vi "Soft_Robot_Model_ffwd.vi"() -> ()   [LabVIEW 2015]
uses:
  <vilib>/addons/Control Design/_Stochastic Systems/Stochastic Systems.llb/Stochastic Systems SubVIs/cd_Stochastic State-Space Model.ctl
  <vilib>/addons/Control Design/_Model Construction/Model Typedefs.llb/CD State Space Model (MIMO).ctl
  <vilib>/addons/Control Design/_Model Construction/Model Typedefs.llb/CD General Elements.ctl
  <vilib>/addons/Control Design/_Stochastic Systems/Stochastic Systems.llb/Stochastic Systems SubVIs/cd_Second-Order Statistics Noise Model.ctl
  <vilib>/Analysis/Matrix/Datatypes/RealMatrix.ctl
  <vilib>/addons/Control Design/_Stochastic Systems/Stochastic Systems.llb/CD CtoD Stochastic Model.ctl
  <vilib>/Analysis/7linalg.llb/Eigenvalue and Vectors Output Option.ctl
  <vilib>/Platform/TimedLoop/XDataNode/timing_clust.ctl
  <vilib>/Platform/TimedLoop/XDataNode/nitl_modes.ctl
  <vilib>/Platform/TimedLoop/XDataNode/wakeup.ctl
  <vilib>/Simulation/Scripting/Companion Diagram/SimConfigNode/SimParams.ctl
  <vilib>/Simulation/Scripting/Companion Diagram/SimConfigNode/_simSolvers.ctl
  <vilib>/Simulation/Implementation/Shared/SIMSCR Execution Mode.ctl
  <vilib>/Simulation/Param Hierarchy/Typedefs/SIMPH Param Control Actions.ctl
  <vilib>/Simulation/Implementation/Shared/NILVSim_ParamChanged.vi
  <vilib>/Simulation/Implementation/Shared/NILVSim_FinishedLate.vi
  <vilib>/Simulation/Implementation/Shared/NILVSIM_BeginStep.vi
  <vilib>/Simulation/SignalArithmetic/Implementation/NILVSim Gain.llb/SIM Gain (scalar).vi
  <vilib>/Simulation/Implementation/Shared/NILVSim_Manager.vi
  <vilib>/Utility/error.llb/Clear Errors.vi
  <vilib>/Simulation/Implementation/Shared/NILVSim_FinalizeModel.vi
  <vilib>/addons/Control Design/_Stochastic Systems/Stochastic Systems.llb/CD Construct Stochastic Model (Numeric).vi
  <vilib>/Analysis/7linalg.llb/Create Special Real Matrix.vi
  <vilib>/addons/Control Design/_Stochastic Systems/Stochastic Systems.llb/CD Construct Noise Model (Numeric).vi
  <vilib>/Analysis/7linalg.llb/Real Eigenvalues and Vectors.vi
  <vilib>/addons/Control Design/_State Feedback Control/State Feedback Control.llb/State Feedback Control SubVis/cd_Linear Quadratic Regulator.vi
  <vilib>/FPGAPlugInAG/myRIO-1900/niLvFpga_Open_myRIO-1900.vi
  <vilib>/rvi/interface/common/dynamic/niFpgaDynamicAddResources.vi
  <vilib>/Utility/error.llb/Error Cluster From Error Code.vi
  <vilib>/rvi/errors/niLvFpgaAdjustHostInterfaceError.vi
  <vilib>/FPGAPlugInAG/Dynamic/niLvFpga_Close_Dynamic.vi
  <vilib>/Simulation/Implementation/Shared/SIM Unbundle Sim Info.vi
  <vilib>/Simulation/Implementation/Shared/SIMSH Read Queue.vi
  <vilib>/Simulation/Implementation/Shared/NILVSim_Initialize.vi
  <vilib>/Utility/file.llb/Write Delimited Spreadsheet.vi
  <vilib>/Utility/file.llb/Write Delimited Spreadsheet (I64).vi
  <vilib>/Utility/file.llb/Write Delimited Spreadsheet (DBL).vi
  <vilib>/addons/Control Design/_Time Response Analysis/Time Response.llb/CD Impulse Response.vi
  <vilib>/addons/Control Design/_Time Response Analysis/Time Response.llb/Time Response subVI/cd_Impulse Response (State-Space).vi
  <vilib>/addons/Control Design/_Time Response Analysis/Time Response.llb/CD Step Response.vi
  <vilib>/addons/Control Design/_Time Response Analysis/Time Response.llb/Time Response subVI/cd_Step Response (State-Space).vi
  <vilib>/Simulation/Utility/Implementation/NILVSim Get Time and IsAcceptedStep.vi
  <vilib>/Simulation/Estimation/Implementation/NILVSim Discrete Kalman Filter.llb/SIM Disc KF Pred and Corr with Pred Gain with Checking Indirect Distributor Sim.vi
  <vilib>/addons/Control Design/_Implementation/CD State Feedback Controller.vi
  <vilib>/addons/Control Design/_Implementation/CD State Feedback Controller (Multiple Outputs).vi
  <vilib>/Simulation/Estimation/Implementation/NILVSim Discrete Kalman Filter.llb/SIM Disc KF Pred and Corr with Pred Gain with Checking Indirect Collector Sim.vi
  <vilib>/Simulation/Implementation/Shared/NILVSim_GetModelError.vi
  <vilib>/Simulation/Implementation/Shared/SIM Bundle Sim Info.vi
  <vilib>/Platform/TimedLoop/XDataNode/XDataNode.xnode
  <vilib>/rvi/interface/nirviOpenFPGA/nirviOpenFPGA.xnode
  FPGA Bitfiles/ACC20115_FPGATarget_CurrentControlle_W-6n2rsGK8k.lvbitx
  Misc/Current Controller.vi
  <vilib>/rvi/interface/nirviReadWriteControl/nirviReadWriteControl.xnode
  <vilib>/rvi/interface/nirviCloseFPGA/nirviCloseFPGA.xnode
  <vilib>/Simulation/Scripting/Companion Diagram/SimConfigNode/SimDog.xnode
  <vilib>/Simulation/Implementation/XNodeFramework/SimXNode/SimX.xnode
  <vilib>/addons/Control Design/_State Feedback Control/NI_CD_State Feedback Control.lvlib
  <vilib>/Analysis/NI_AALPro.lvlib
  <vilib>/Platform/TimedLoop/XDataNode/XDNodeRunTimeDep.lvlib
  <vilib>/rvi/interface/Simulation/niFpgaSimulationCallBeginRW.vi
  <vilib>/addons/Control Design/_Stochastic Systems/NI_CD_Stochastic Systems.lvlib
  <vilib>/addons/Control Design/_State-Space Analysis/NI_CD_State-Space Analysis.lvlib
  NiFpgaLv.dll
  <vilib>/addons/Control Design/_Implementation/NI_CD_Implementation.lvlib
  <vilib>/addons/Control Design/_Time Response Analysis/NI_CD_Time Response.lvlib
  <vilib>/Simulation/Estimation/Implementation/NILVSim Discrete Kalman Filter.llb/SIM Disc KF Pred and Corr with Pred Gain with Checking Indirect Sim.vi
  <vilib>/Simulation/Implementation/Shared/NI_SIM_Implementation.lvlib
  <vilib>/addons/Control Design/_Model Construction/NI_LinSys_Model Typedefs.lvlib
  <vilib>/Analysis/Matrix/NI_Matrix.lvlib
panel:
  out "Error":errorcluster
  in  "Tab Control":T1(tab)
  out "Valve Current (mA)":dbl(graph)
  out "Kinect Fusion":dbl(graph)
  in  "Current (mA)":i32
  out "Plant Output and KF estimation":dbl[][](graph)=[[694.135, 693.2125685090368]]
  out "KF Predictor Gain L(k)":dbl[][](array[numeric])=[[1.0]] format="%#.6g"
  out "KF Gain M(k)":dbl[][](array[numeric]) format="%#.6g"
  in  "Stop":bool
  out "LQR Eigenvalues":cdb[](array[numeric]) format="%.5f"
  out "P(k+1|k)":dbl[][](array[numeric])
  out "P(k|k)":dbl[][](array[numeric])
  out "LQR Q Eig Vals":cdb[](array[numeric])
  out "LQR R Eig Val":cdb[](array[numeric])
  out "Optimal LQR Gains":dbl[][](array[numeric])
  out "Control Action":dbl
  out "Controllable?":bool
  out "Stable?":bool
  out "Detectable?":bool
  out "Observable?":bool
  out "LQR Q Matrix":T2
  out "LQR R Matrix":T2
  out "FPGA Overflow?":bool
  in  "SP (mm)":dbl(knob)=641.7660208643815 scale=670.0..695.0
  out "Local Kalman Filters & Central Site Fusion":dbl[][](graph)
  out "Stochastic SS Model":T3={"Sampling Time (s)"=0.0, "G"=[], "B"=[[-1.71e-07], [6.47e-07]], "A"=[], "C"=[], "D"=[], "H"=[]} {"H" format="%#.2g"; "D" format="%#.2g"; "C" format="%#.2g"; "A" format="%#.2g"; "B" format="%#.2g"; "G" format="%#.2g"; "Sampling Time (s)" format="%.2f"}
  out "Deterministic SS Model":T4={"properties"={"Model name"="", "Input names"=[], "Output names"=[], "Input Delays"=[], "Output Delays"=[], "Sampling Time"=0.0, "Notes"=""}, "A"=[], "B"=[[-1.706e-07], [6.469e-07]], "C"=[], "D"=[], "StateNames"=[], "Transport Delay"=[]} {"Transport Delay" format="%.2f"; "D" format="%#.2g"; "C" format="%#.2g"; "B" format="%#.2g"; "A" format="%#.2g"; "properties"."Sampling Time" format="%#.6p"; "properties"."Output Delays" format="%.4f"; "properties"."Input Delays" format="%.4f"}
  out "DAC Loop Error":errorcluster
  out "LQR Error":errorcluster
  out "KF Noise Model":T6 {"N" format="%#.2g"; "R" format="%#.2g"; "E{v}" format="%#.2g"; "E{w}" format="%#.2g"; "Q" format="%#.2g"}
  out "FPGA Loop Error":errorcluster
  out "KF Model Error":errorcluster
  out "UDP Loop Error":errorcluster
  out "Step Response Graph":cluster{"time":dbl[], dbl[]}[](graph)=[{"time"=[0.0, 0.1, 0.2, 0.30000000000000004, 0.4, 0.5, 0.6000000000000001, 0.7000000000000001, 0.8, 0.9, 1.0, 1.1, 1.2000000000000002, 1.3, 1.4000000000000001, 1.5, 1.6, 1.7000000000000002, 1.8, 1.9000000000000001, 2.0, 2.1, 2.2, 2.3000000000000003, 2.4000000000000004, 2.5, 2.6, 2.7, 2.8000000000000003, 2.9000000000000004, 3.0, 3.1, 3.2, 3.3000000000000003, 3.4000000000000004, 3.5, 3.6, 3.7, 3.8000000000000003, 3.9000000000000004, 4.0, 4.1000000000000005, 4.2, 4.3, 4.4, 4.5, 4.6000000000000005, 4.7, 4.800000000000001, 4.9, 5.0, 5.1000000000000005, 5.2, 5.300000000000001, 5.4, 5.5, 5.6000000000000005, 5.7, 5.800000000000001, 5.9, 6.0, 6.1000000000000005, 6.2, 6.300000000000001, 6.4, 6.5, 6.6000000000000005, 6.7, 6.800000000000001, 6.9, 7.0, 7.1000000000000005, 7.2, 7.300000000000001, 7.4, 7.5, 7.6000000000000005, 7.7, 7.800000000000001, 7.9, 8.0], [0.0, 0.0004663473208612627, 0.0017296930483795164, 0.0035885524413313812, 0.00585108885158747, 0.008342022204108804, 0.010907538001557412, 0.013418337758795643, 0.01577103010603519, 0.017888100567384182, 0.019716719021094366, 0.02122664935211373, 0.022407518377011763, 0.02326568343598631, 0.02382091276348735, 0.024103062386256875, 0.024148900146291487, 0.023999193507947617, 0.02369614475738421, 0.023281226369499006, 0.02279344169187109, 0.022268012342287972, 0.021735474206151545, 0.021221148763839872, 0.020744945570676618, 0.020321444775591793, 0.01996020519209235, 0.019666243132932183, 0.01944062944497821, 0.019281156374667745, 0.019183031510994153, 0.01913956258079366, 0.019142803850451515, 0.019184141922185993, 0.01925480547445023, 0.01934628972900578, 0.019450691946355205, 0.019560958936806403, 0.019671051366119408, 0.01977603252338114, 0.019872091237783975, 0.01995650984687708, 0.020027588622327185, 0.02008453795668775, 0.020127349020610013, 0.02015665263024424, 0.020173574831124263, 0.02017959631108057, 0.02017642129264157, 0.02016586010332895, 0.020149728243942358, 0.02012976351919565, 0.020107561696361465, 0.0200845302370225, 0.0200618589138676, 0.02004050557782586, 0.020021194971562285, 0.020004428277976674, 0.01999050102686616, 0.019979527036564866, 0.0199714662161444, 0.019966154273690646, 0.019963332644441115, 0.019962677248304108, 0.019963824991160707, 0.019966397222957007, 0.019970019645588307, 0.019974338415697335, 0.019979032405429503, 0.019983821764274674, 0.01998847306610796, 0.01999280142814749, 0.019996670055101227, 0.019999987695808956, 0.020002704505559007, 0.020004806789810977, 0.02000631106930135, 0.020007257857379883, 0.020007705482562522, 0.0200077242268862, 0.02000739098734998]}]
  out "Impulse Response":cluster{"time":dbl[], dbl[]}[](graph)=[{"time"=[0.0, 0.1, 0.2, 0.30000000000000004, 0.4, 0.5, 0.6000000000000001, 0.7000000000000001, 0.8, 0.9, 1.0, 1.1, 1.2000000000000002, 1.3, 1.4000000000000001, 1.5, 1.6, 1.7000000000000002, 1.8, 1.9000000000000001, 2.0, 2.1, 2.2, 2.3000000000000003, 2.4000000000000004, 2.5, 2.6, 2.7, 2.8000000000000003, 2.9000000000000004, 3.0, 3.1, 3.2, 3.3000000000000003, 3.4000000000000004, 3.5, 3.6, 3.7, 3.8000000000000003, 3.9000000000000004, 4.0, 4.1000000000000005, 4.2, 4.3, 4.4, 4.5, 4.6000000000000005, 4.7, 4.800000000000001, 4.9, 5.0, 5.1000000000000005, 5.2, 5.300000000000001, 5.4, 5.5, 5.6000000000000005, 5.7, 5.800000000000001, 5.9, 6.0, 6.1000000000000005, 6.2, 6.300000000000001, 6.4, 6.5, 6.6000000000000005, 6.7, 6.800000000000001, 6.9, 7.0, 7.1000000000000005, 7.2, 7.300000000000001, 7.4, 7.5, 7.6000000000000005, 7.7, 7.800000000000001, 7.9, 8.0], [0.0, 0.008988172215977587, 0.015941438633037666, 0.02091487162309135, 0.024042908393783827, 0.02551889757722494, 0.02557569478365717, 0.024467992676866855, 0.022456868580669295, 0.019796844996257237, 0.016725591461953054, 0.013456253705261323, 0.010172280017081137, 0.007024525658691236, 0.004130353039235721, 0.0015744064999214857, -0.0005892768149515742, -0.002334157452931432, -0.0036574068645988137, -0.004575736995437892, -0.005121104002831364, -0.005336502802076594, -0.005272025764550862, -0.004981315552097141, -0.004518500722641401, -0.003935664888301879, -0.0032808669235171064, -0.0025967016806585676, -0.001919368189106927, -0.0012781953978247278, -0.0006955639255905182, -0.0001871555662120171, 0.0002375401230830873, 0.0005745316131444697, 0.0008245089129275849, 0.0009919638112413014, 0.0010842980213564997, 0.0011109616697939839, 0.0010826555079039139, 0.0010106212985917036, 0.0009060364188353945, 0.0007795211078167689, 0.000640760178844977, 0.0004982355180431294, 0.00035906135961267507, 0.00022891114129368586, 0.0001120226402826769, 1.1266967989904443e-05, -7.17332656671379e-05, -0.00013645086398689086, -0.0001832792705777772, -0.0002133479298936649, -0.00022833790229576505, -0.0002303060085980187, -0.00022152389413133484, -0.00020433657074322872, -0.00018104328983030286, -0.0001538020745465803, -0.00012455793086593947, -9.499368500849999e-05, -6.650156442132397e-05, -4.0173044664881016e-05, -1.6804109357439747e-05, 3.087108111676786e-06, 1.9233341685522883e-05, 3.158477953815003e-05, 4.027189426429472e-05, 4.556687476968165e-05, 4.7845653868121716e-05, 4.755213725597536e-05, 4.516584913005334e-05, 4.117383523520003e-05, 3.6047319585871326e-05, 3.0223306623967816e-05, 2.4091062632339335e-05, 1.7983202024296476e-05, 1.2170946052935176e-05, 6.863011578249593e-06, 2.207522022942255e-06, -1.7036935523276584e-06, -4.8290401595337954e-06]}]
  out "Step and Impulse Response Plots":cluster{"time":dbl[], dbl[]}[](graph)=[{"time"=[0.0, 0.1, 0.2, 0.30000000000000004, 0.4, 0.5, 0.6000000000000001, 0.7000000000000001, 0.8, 0.9, 1.0, 1.1, 1.2000000000000002, 1.3, 1.4000000000000001, 1.5, 1.6, 1.7000000000000002, 1.8, 1.9000000000000001, 2.0, 2.1, 2.2, 2.3000000000000003, 2.4000000000000004, 2.5, 2.6, 2.7, 2.8000000000000003, 2.9000000000000004, 3.0, 3.1, 3.2, 3.3000000000000003, 3.4000000000000004, 3.5, 3.6, 3.7, 3.8000000000000003, 3.9000000000000004, 4.0, 4.1000000000000005, 4.2, 4.3, 4.4, 4.5, 4.6000000000000005, 4.7, 4.800000000000001, 4.9, 5.0, 5.1000000000000005, 5.2, 5.300000000000001, 5.4, 5.5, 5.6000000000000005, 5.7, 5.800000000000001, 5.9, 6.0, 6.1000000000000005, 6.2, 6.300000000000001, 6.4, 6.5, 6.6000000000000005, 6.7, 6.800000000000001, 6.9, 7.0, 7.1000000000000005, 7.2, 7.300000000000001, 7.4, 7.5, 7.6000000000000005, 7.7, 7.800000000000001, 7.9, 8.0], [0.0, 0.0004663473208612627, 0.0017296930483795164, 0.0035885524413313812, 0.00585108885158747, 0.008342022204108804, 0.010907538001557412, 0.013418337758795643, 0.01577103010603519, 0.017888100567384182, 0.019716719021094366, 0.02122664935211373, 0.022407518377011763, 0.02326568343598631, 0.02382091276348735, 0.024103062386256875, 0.024148900146291487, 0.023999193507947617, 0.02369614475738421, 0.023281226369499006, 0.02279344169187109, 0.022268012342287972, 0.021735474206151545, 0.021221148763839872, 0.020744945570676618, 0.020321444775591793, 0.01996020519209235, 0.019666243132932183, 0.01944062944497821, 0.019281156374667745, 0.019183031510994153, 0.01913956258079366, 0.019142803850451515, 0.019184141922185993, 0.01925480547445023, 0.01934628972900578, 0.019450691946355205, 0.019560958936806403, 0.019671051366119408, 0.01977603252338114, 0.019872091237783975, 0.01995650984687708, 0.020027588622327185, 0.02008453795668775, 0.020127349020610013, 0.02015665263024424, 0.020173574831124263, 0.02017959631108057, 0.02017642129264157, 0.02016586010332895, 0.020149728243942358, 0.02012976351919565, 0.020107561696361465, 0.0200845302370225, 0.0200618589138676, 0.02004050557782586, 0.020021194971562285, 0.020004428277976674, 0.01999050102686616, 0.019979527036564866, 0.0199714662161444, 0.019966154273690646, 0.019963332644441115, 0.019962677248304108, 0.019963824991160707, 0.019966397222957007, 0.019970019645588307, 0.019974338415697335, 0.019979032405429503, 0.019983821764274674, 0.01998847306610796, 0.01999280142814749, 0.019996670055101227, 0.019999987695808956, 0.020002704505559007, 0.020004806789810977, 0.02000631106930135, 0.020007257857379883, 0.020007705482562522, 0.0200077242268862, 0.02000739098734998]}, {"time"=[0.0, 0.1, 0.2, 0.30000000000000004, 0.4, 0.5, 0.6000000000000001, 0.7000000000000001, 0.8, 0.9, 1.0, 1.1, 1.2000000000000002, 1.3, 1.4000000000000001, 1.5, 1.6, 1.7000000000000002, 1.8, 1.9000000000000001, 2.0, 2.1, 2.2, 2.3000000000000003, 2.4000000000000004, 2.5, 2.6, 2.7, 2.8000000000000003, 2.9000000000000004, 3.0, 3.1, 3.2, 3.3000000000000003, 3.4000000000000004, 3.5, 3.6, 3.7, 3.8000000000000003, 3.9000000000000004, 4.0, 4.1000000000000005, 4.2, 4.3, 4.4, 4.5, 4.6000000000000005, 4.7, 4.800000000000001, 4.9, 5.0, 5.1000000000000005, 5.2, 5.300000000000001, 5.4, 5.5, 5.6000000000000005, 5.7, 5.800000000000001, 5.9, 6.0, 6.1000000000000005, 6.2, 6.300000000000001, 6.4, 6.5, 6.6000000000000005, 6.7, 6.800000000000001, 6.9, 7.0, 7.1000000000000005, 7.2, 7.300000000000001, 7.4, 7.5, 7.6000000000000005, 7.7, 7.800000000000001, 7.9, 8.0], [0.0, 0.008988172215977587, 0.015941438633037666, 0.02091487162309135, 0.024042908393783827, 0.02551889757722494, 0.02557569478365717, 0.024467992676866855, 0.022456868580669295, 0.019796844996257237, 0.016725591461953054, 0.013456253705261323, 0.010172280017081137, 0.007024525658691236, 0.004130353039235721, 0.0015744064999214857, -0.0005892768149515742, -0.002334157452931432, -0.0036574068645988137, -0.004575736995437892, -0.005121104002831364, -0.005336502802076594, -0.005272025764550862, -0.004981315552097141, -0.004518500722641401, -0.003935664888301879, -0.0032808669235171064, -0.0025967016806585676, -0.001919368189106927, -0.0012781953978247278, -0.0006955639255905182, -0.0001871555662120171, 0.0002375401230830873, 0.0005745316131444697, 0.0008245089129275849, 0.0009919638112413014, 0.0010842980213564997, 0.0011109616697939839, 0.0010826555079039139, 0.0010106212985917036, 0.0009060364188353945, 0.0007795211078167689, 0.000640760178844977, 0.0004982355180431294, 0.00035906135961267507, 0.00022891114129368586, 0.0001120226402826769, 1.1266967989904443e-05, -7.17332656671379e-05, -0.00013645086398689086, -0.0001832792705777772, -0.0002133479298936649, -0.00022833790229576505, -0.0002303060085980187, -0.00022152389413133484, -0.00020433657074322872, -0.00018104328983030286, -0.0001538020745465803, -0.00012455793086593947, -9.499368500849999e-05, -6.650156442132397e-05, -4.0173044664881016e-05, -1.6804109357439747e-05, 3.087108111676786e-06, 1.9233341685522883e-05, 3.158477953815003e-05, 4.027189426429472e-05, 4.556687476968165e-05, 4.7845653868121716e-05, 4.755213725597536e-05, 4.516584913005334e-05, 4.117383523520003e-05, 3.6047319585871326e-05, 3.0223306623967816e-05, 2.4091062632339335e-05, 1.7983202024296476e-05, 1.2170946052935176e-05, 6.863011578249593e-06, 2.207522022942255e-06, -1.7036935523276584e-06, -4.8290401595337954e-06]}]
  in  "A":dbl[][](array[numeric])=[[-0.275, -0.05848], [0.3155, 0.05955]] format="%#.5g"
  in  "B":dbl[][](array[numeric])=[[-0.0001629], [8.009e-05]] format="%#.5g"
  in  "C":dbl[][](array[numeric])=[[0.742, 2.316]] format="%#.5g"
  in  "G":dbl[][](array[numeric])=[[0.7998], [2.296]] format="%#.2g"
  in  "xhat(0|-1)":dbl[](array[numeric])=[687.0, 687.0]
  in  "P(0|-1)":dbl[][](array[numeric])=[[1.0, 0.0], [0.0, 1.0]]
  in  "KF R":dbl[](array[slide])=[0.013076604860118303] scale=0.001..5000.0
  in  "KF Q":dbl[](array[slide])=[0.44512793318037663] scale=0.01..100.0
  in  "yhat(KT)":path=path "c:/LQGyhat.csv"
  in  "input":path=path "c:/current.csv"
  in  "y(kT)":path=path "c:/Fusionyhat.csv"
  in  "SP":path=path "c:/setpoint.csv"
  in  "LQR R":dbl[](array[knob]) scale=1.0..2.0
  in  "LQR Matrix (Q)":dbl[](array[knob]) scale=0.0..9.0
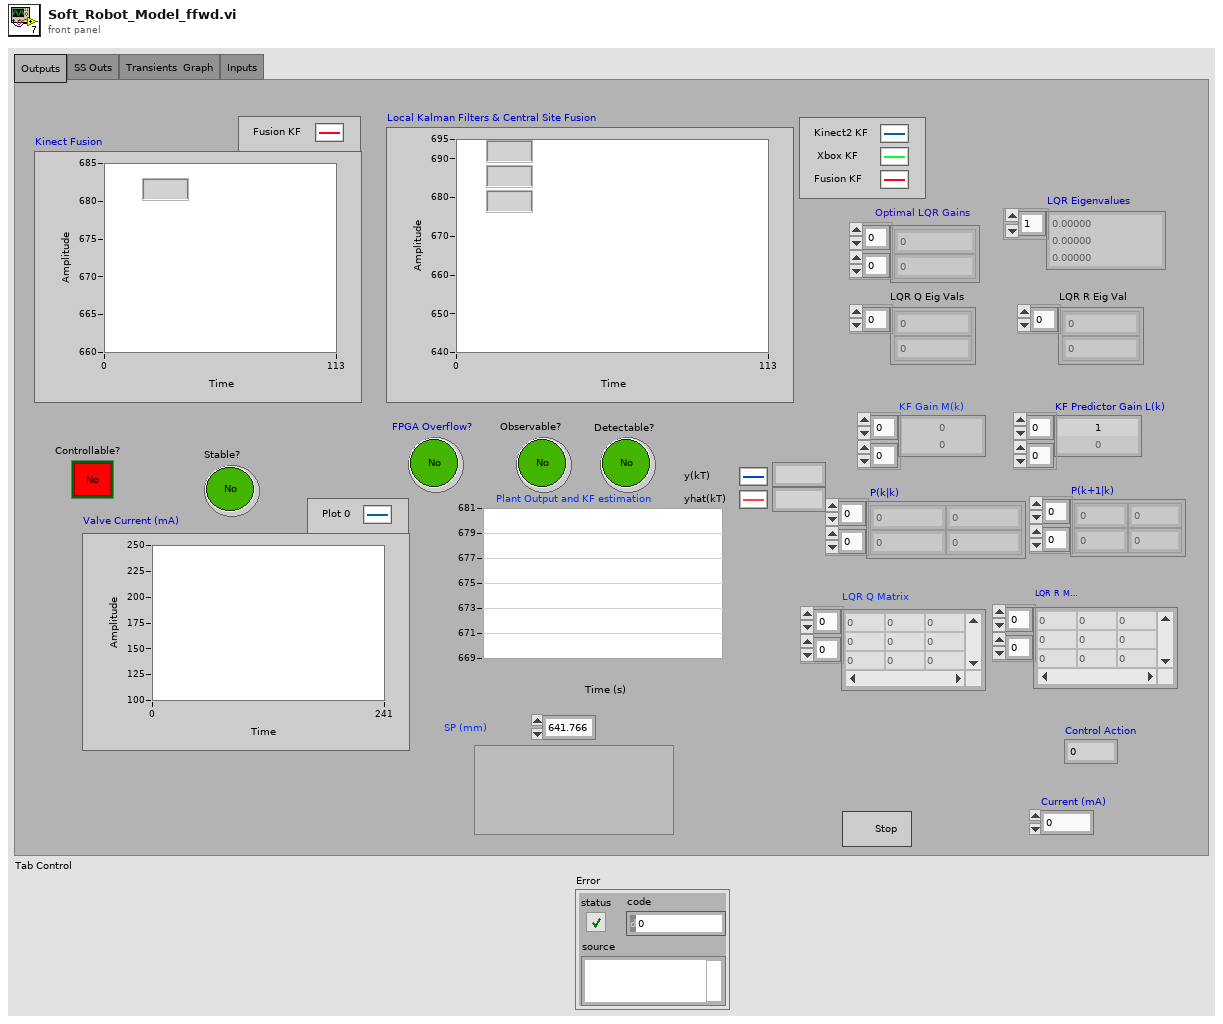
[diagram p1: front panel]
types:
  T1 = enum32{"Outputs", "SS Outs", "Transients  Graph", "Inputs"}
  T2 = typedef "NI_Matrix.lvlib/RealMatrix.ctl" = dbl[][]
  T3 = typedef "NI_CD_Stochastic Systems.lvlib/cd_Stochastic State-Space Model.ctl" = cluster{"Sampling Time (s)":dbl, "G":dbl[][], "B":dbl[][], "A":dbl[][], "C":dbl[][], "D":dbl[][], "H":dbl[][]}
  T4 = typedef "NI_LinSys_Model Typedefs.lvlib/CD State Space Model (MIMO).ctl" = cluster{"properties":T5, "A":dbl[][], "B":dbl[][], "C":dbl[][], "D":dbl[][], "StateNames":string[], "Transport Delay":dbl[][]}
  T5 = typedef "NI_LinSys_Model Typedefs.lvlib/CD General Elements.ctl" = cluster{"Model name":string, "Input names":string[], "Output names":string[], "Input Delays":dbl[], "Output Delays":dbl[], "Sampling Time":dbl, "Notes":string}
  T6 = typedef "NI_CD_Stochastic Systems.lvlib/cd_Second-Order Statistics Noise Model.ctl" = cluster{"Q":dbl[][], "E{w}":dbl[], "E{v}":dbl[], "R":dbl[][], "N":dbl[][]}
  T7 = typedef "NI_AALPro.lvlib/Eigenvalue and Vectors Output Option.ctl" = i32
  T8 = enum32{"Identity", "Diagonal", "Toepliz", "Vandermonde", "Companion"}
  T9 = typedef "NI_CD_Stochastic Systems.lvlib/CD CtoD Stochastic Model.ctl" = enum16{"Truncation of Taylor Series", "Numerical Integration"}
  T10 = enum16{"state weighting", "output weighting, Dim Q = Ny", "output weighting, Dim Q = Nx"}
  T11 = typedef "XDNodeRunTimeDep.lvlib/timing_clust.ctl" = cluster{"Expected End [f-1]":u64, "Actual End [f-1]":u64, "Finished Late? [f-1]":bool, "Expected End [i-1]":u64, "Actual End [i-1]":u64, "Finished Late? [i-1]":bool, "Expected Start [i]":u64, "Actual Start [i]":u64, "Expected Start [f]":u64, "Actual Start [f]":u64, "Source Name":string, "Structure Name":string, "Period":i64, "Deadline":i64, "Offset":i64, "Start":i64, "Priority":i32, "Timeout":i32, "Mode":T12, "Wakeup Reason":T13, "Error":errorcluster, "Source Type":string, "Secondary Source Type":string, "Global End Time":u64, "Global Start Time":u64, "Frame Duration":u64, "Iteration Duration":u64, "Assigned CPU":i32, "I/O Scan Engine Mode":u32}
  T12 = typedef "XDNodeRunTimeDep.lvlib/nitl_modes.ctl" = enum32{"No Change", "Process missed periods, maintain original phase", "Discard missed periods, maintain original phase", "Process missed periods, ignore original phase", "Discard missed periods, ignore original phase"}
  T13 = typedef "XDNodeRunTimeDep.lvlib/wakeup.ctl" = enum32{"Normal", "Aborted", "Asynchronous wakeup", "Timing source error", "Timed loop error", "Timeout"}
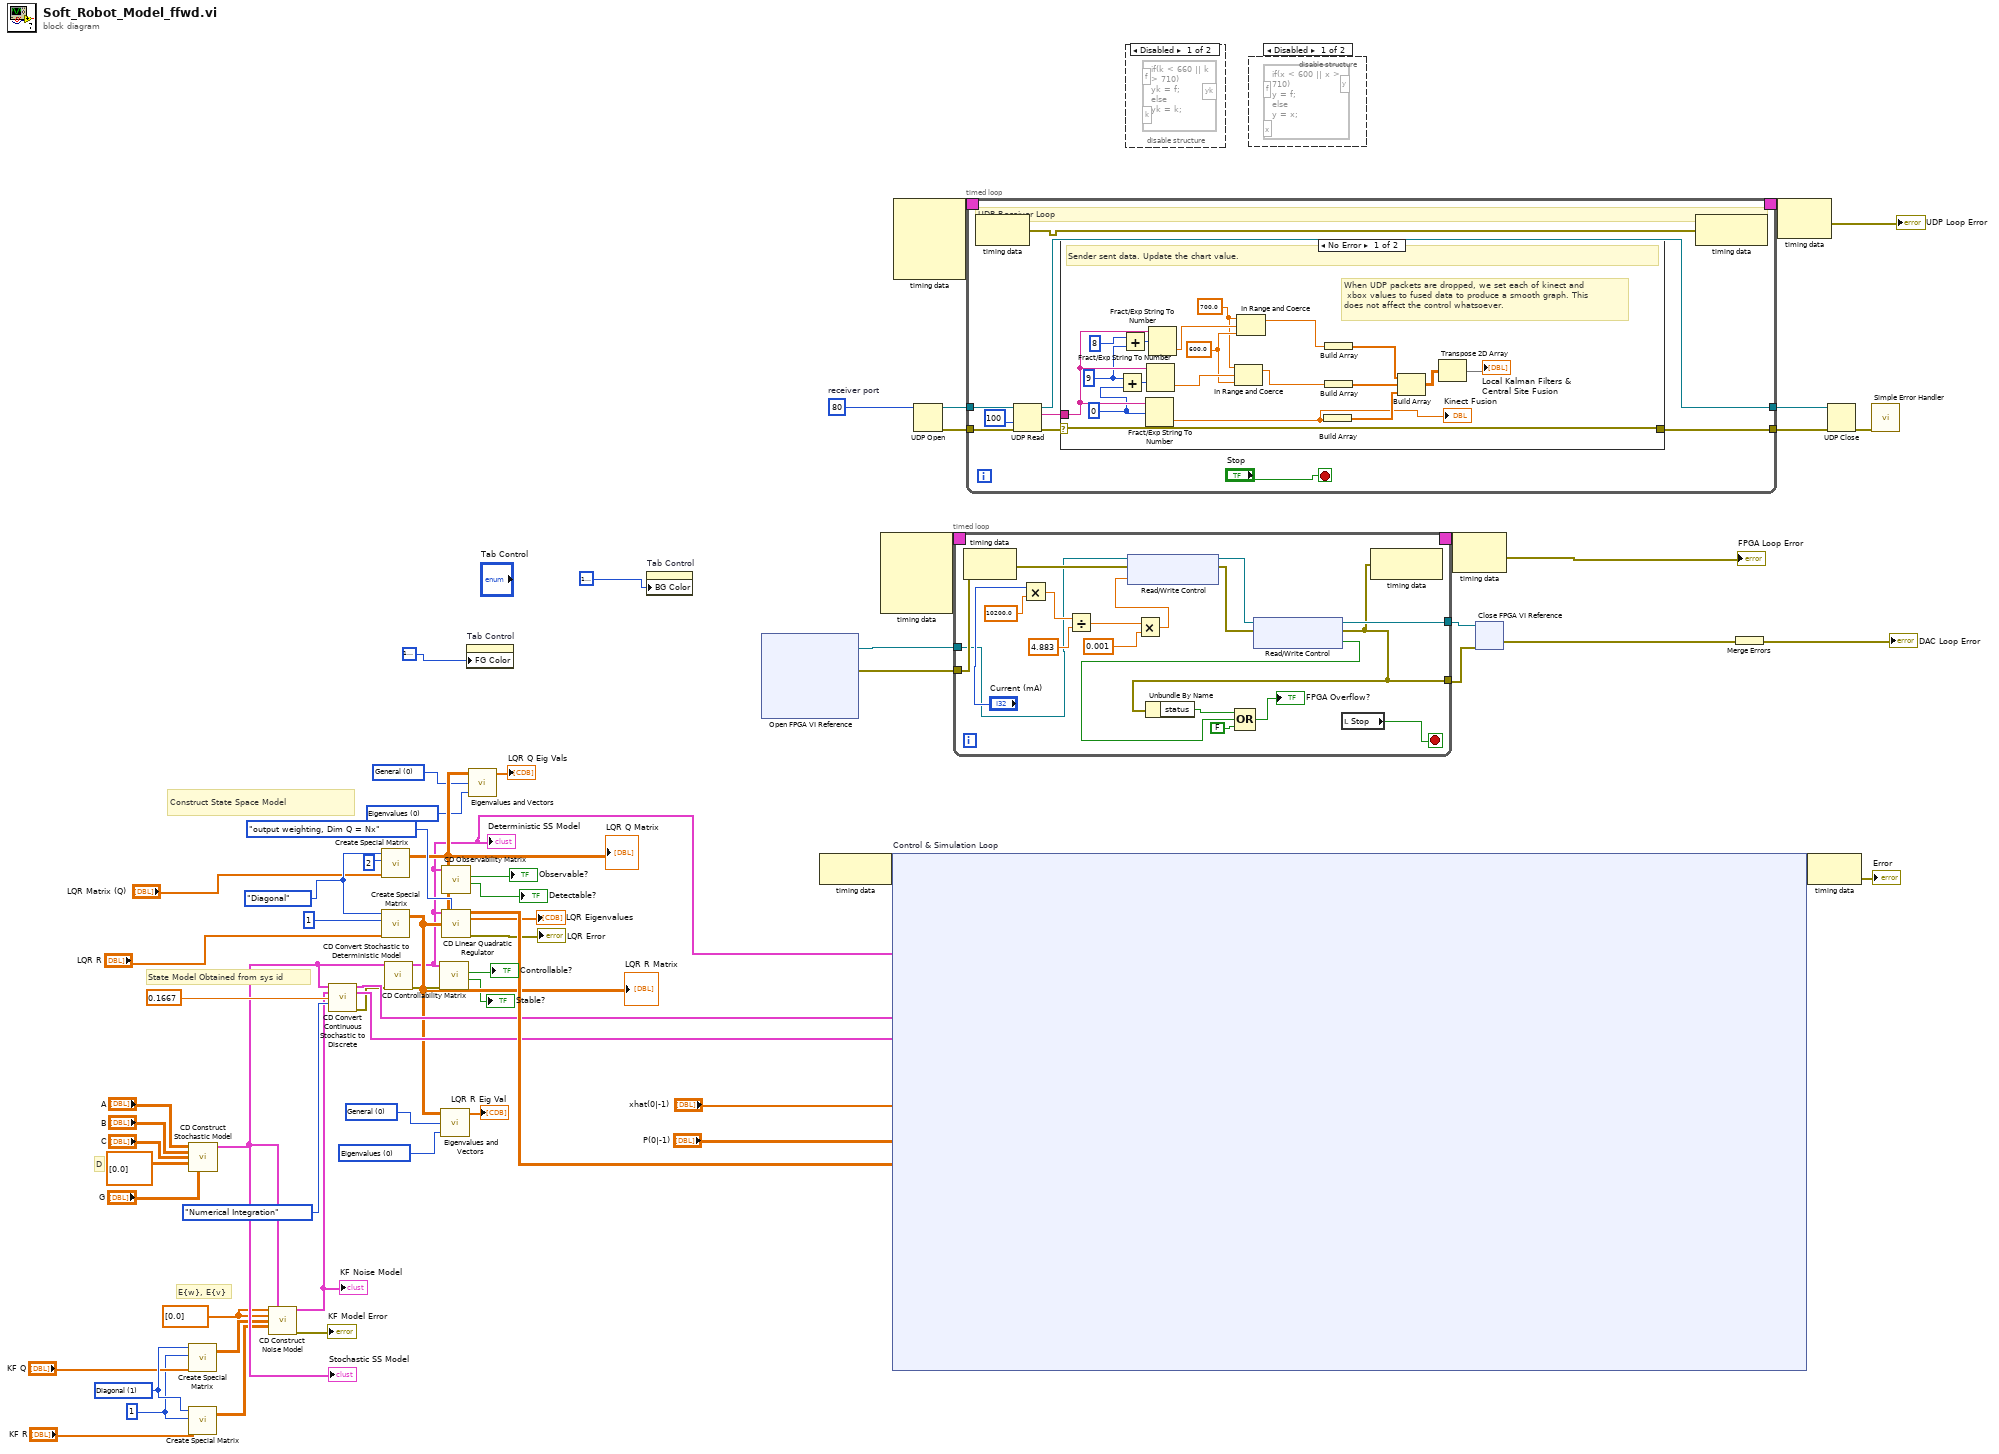
[diagram p0: block diagram]
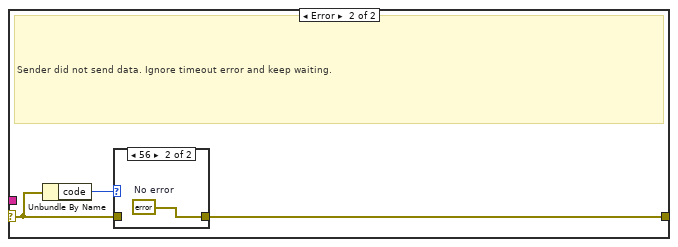
[diagram p4: hidden frame]
diagram:
  w17 = T7 0 items=["Eigenvalues", "Eigenvalues & Vectors"] ("output option")
  w18 = 0 items=["General", "Symmetric"] ("matrix type")
  w20 = T7 0 items=["Eigenvalues", "Eigenvalues & Vectors"] ("output option")
  w21 = 0 items=["General", "Symmetric"] ("matrix type")
  w25 = T8."Diagonal" ("matrix type")
  w26 = 1 ("KF Q/R Size")
  w30 = dbl[] [0.0] ("E{w}")
  w31 = 1 items=["Identity", "Diagonal", "Toeplitz", "Vandermonde", "Companion", "Hankel", "Hadamard", "Wilkinson", "Hilbert", "Inverse Hilbert", "Rosser", "Pascal"] ("matrix type")
  w56 = u16 80  # receiver port
  # "E{w}, E{v}"
  # "D"
  # "State Model Obtained from sys id"
  # "Construct State Space Model"
  n1 = call-poly <vilib>:"Create Special Matrix.vi"("matrix type"=w31, "matrix size"=w26, "Input Vector1"="KF Q") -> ("Special Matrix"=w33:T2)  [unwired: 2 in, 1 out]
  n2 = call-poly <vilib>:"Create Special Matrix.vi"("matrix type"=w31, "matrix size"=w26, "Input Vector1"="KF R") -> ("Special Matrix"=w32:T2)  [unwired: 2 in, 1 out]
  n3 = call-poly <vilib>:"CD Construct Stochastic Model.vi"("A"="A", "B"="B", "C"="C", "D"=dbl[][] [[0.0]], "G"="G") -> ("Stochastic State-Space Model"=w40:T3)  [unwired: 3 in, 7 out]
  "Stochastic SS Model" <- w40
  n4 = call-poly <vilib>:"CD Construct Noise Model.vi"("E{w}"=w30, "Stochastic State-Space Model"=w40, "E{v}"=w30, "Q"=w33, "R"=w32) -> ("Second-Order Statistics Noise Model out"=w41:T6, "error out"=→"KF Model Error":errorcluster)  [unwired: 2 in, 7 out]
  "KF Noise Model" <- w41
  n5 = call <vilib>:"CD Convert Continuous Stochastic to Discrete.vi"("Continuous Stochastic\nState-Space Model"=w40, "Continuous Second-Order\nStatistics Noise Model"=w41, "Sampling Time (s)"=0.1667, "Method"=CD_CtoD_Stochastic_Model."Numerical Integration") -> ("Discrete Stochastic\nState-Space Model"=w50:T3, "Discrete Second-Order\nStatistics Noise Model"=w51:T6, "error out"=w39:errorcluster)  [unwired: 1 in, 8 out]
  n6 = call-poly <vilib>:"Create Special Matrix.vi"("matrix type"=w25, "matrix size"=2, "Input Vector1"="LQR Matrix (Q)") -> ("Special Matrix"=w22:T2)  [unwired: 2 in, 1 out]
  "LQR Q Matrix" <- w22
  n7 = call-poly <vilib>:"Create Special Matrix.vi"("matrix type"=w25, "matrix size"=1, "Input Vector1"="LQR R") -> ("Special Matrix"=w15:T2)  [unwired: 2 in, 1 out]
  "LQR R Matrix" <- w15
  n8 = call <vilib>:"CD Convert Stochastic to Deterministic Model.vi"("Stochastic State-Space Model"=w40, "error in (no error)"=w39) -> ("Deterministic State-Space Model"=w10:T4, "error out"=w38:errorcluster)  [unwired: 12 in]
  "Deterministic SS Model" <- w10
  n9 = call <vilib>:"CD Controllability Matrix.vi"("error in (no error)"=w38, "State-Space Model"=w10) -> ("Is Stabilizable?"=→"Stable?":bool, "Is Controllable?"=→"Controllable?":bool)  [unwired: 6 in, 2 out]
  n10 = call-poly <vilib>:"Eigenvalues and Vectors.vi"("output option"=w17, "matrix type"=w18, "Input Matrix"=w15) -> ("Eigenvalues"=→"LQR R Eig Val":cdb[])  [unwired: 2 out]
  n11 = call <vilib>:"CD Observability Matrix.vi"("State-Space Model"=w10) -> ("Is Detectable?"=→"Detectable?":bool, "Is Observable?"=→"Observable?":bool)  [unwired: 7 in, 2 out]
  n12 = call-poly <vilib>:"CD Linear Quadratic Regulator.vi"("State-Space Model"=w10, "Weighting Type"=T10."output weighting, Dim Q = Nx", "Q"=w22, "R"=w15) -> ("Optimal Gain (K)"=w52:dbl[][], "Eigenvalues"=→"LQR Eigenvalues":cdb[], "error out"=→"LQR Error":errorcluster)  [unwired: 8 in, 1 out]
  n13 = property on="Tab Control" class="TabCtl (strict)"("FG Color"=u32 16777226) -> ()  [unwired: 2 in, 2 out]
  n14 = call-poly <vilib>:"Eigenvalues and Vectors.vi"("output option"=w20, "matrix type"=w21, "Input Matrix"=w22) -> ("Eigenvalues"=→"LQR Q Eig Vals":cdb[])  [unwired: 2 out]
  n15 = property on="Tab Control" class="TabCtl (strict)"("BG Color"=u32 16777226) -> ()  [unwired: 2 in, 2 out]
  n16 = xnode "Open FPGA VI Reference"() -> ("FPGA VI Reference Out"=w7:refnum<k20>, "error out"=w6:errorcluster)  [unwired: 2 in]
  n17 = node-c288() -> (w3:variant)  [unwired: 1 in]
  n18 = node-c288() -> (w66:T11)  [unwired: 4 in]
  n19 = node-c254 "Control & Simulation Loop"(w3, w51, "xhat(0|-1)", "P(0|-1)", w50, w10, w52) -> (w2:variant)
  n20 = node-c288() -> (w55:T11)  [unwired: 4 in]
  n21 = UDP Open(11:w56) -> (port=w57:refnum<k16>, 0:w58:errorcluster)  [unwired: 4 in, 1 out]
  n22 = timed-loop {
    tunnel: w6 -> [w73]
    tunnel: [w72] -> w64
    tunnel: [w81] -> w68
    timing: w66 -> [_]
    timing-out: [_] -> w65
    tunnel: w7 -> [w71]
    stop <- w70 stop-if-true
    n23 = node-c288() -> ()  [unwired: 1 in, 1 out]
    n24 = Multiply(x="Current (mA)", y=10200.0) -> (x*y=w76:dbl)
    n25 = Divide(x=w76, y=4.883) -> (x/y=w79:dbl)
    n26 = Multiply(x=w79, y=0.001) -> (x*y=w75:dbl)
    n27 = xnode "Read/Write Control"("FPGA VI Reference In"=w71, "error in"=w73, "DAC Inlet Valve"=w75) -> ("FPGA VI Reference Out"=w86:refnum<k20>, "error out"=w85:errorcluster)
    n28 = xnode "Read/Write Control"("FPGA VI Reference In"=w86, "error in"=w85) -> ("FPGA VI Reference Out"=w81:refnum<k20>, "error out"=w72:errorcluster, "Inlet Overflow?"=w82:bool)
    n29 = Unbundle By Name(w72) -> ("status"=w83:bool)
    n30 = Compound Arithmetic op=OR(w83, w82, FALSE ("value")) -> (→"FPGA Overflow?":bool)
    n31 = local read "Stop"() -> (w70:bool)
    n32 = node-c288(w72) -> ()  [unwired: 1 out]
  }
  n33 = timed-loop {
    tunnel: w57 -> [w99]
    tunnel: [w93] -> w61
    tunnel: w58 -> [w98]
    tunnel: [w94] -> w59
    timing: w55 -> [_]
    timing-out: [_] -> w54
    stop <- "Stop" stop-if-true
    # "UDP Receiver Loop"
    n34 = node-c288() -> (w91:errorcluster)  [unwired: 1 in]
    n35 = UDP Read(connection ID=w99, timeout ms (25000)=100, 8:w98) -> (data out=w96:string, error out=w95:errorcluster, 3:w93:refnum<k16>)  [unwired: 3 out]
    n36 = case shown="No Error" w95 {
      selector: w95 -> [w123 w125]
      tunnel: w96 -> [w122 _]
      tunnel: [w123 w124] -> w94
      frame No Error {
        w106 = 600.0 ("lower limit")
        w105 = 700.0 ("upper limit")
        w118 = 9 ("x")
        w120 = 0 ("offset")
        # "When UDP packets are dropped, we set each of kinect and\n xbox values to fused data to produce a smooth graph. This does not affect the control whatsoever."
        # "Sender sent data. Update the chart value."
        n37 = Add(x=w118, y=w120) -> (x+y=w121:i32)
        n38 = Add(x=8, y=w118) -> (x+y=w119:i32)
        n39 = Fract/Exp String To Number(string=w122, offset=w120) -> (number=w111:dbl)  [unwired: 2 in, 1 out]
        "Kinect Fusion" <- w111
        n40 = Fract/Exp String To Number(string=w122, offset=w121) -> (number=w107:dbl)  [unwired: 2 in, 1 out]
        n41 = Fract/Exp String To Number(string=w122, offset=w119) -> (number=w110:dbl)  [unwired: 2 in, 1 out]
        n42 = In Range and Coerce(upper limit=w105, x=w107, lower limit=w106) -> (coerced(x)=w108:dbl)  [unwired: 1 out]
        n43 = In Range and Coerce(upper limit=w105, x=w110, lower limit=w106) -> (coerced(x)=w109:dbl)  [unwired: 1 out]
        n44 = Build Array(w111) -> (w115:dbl[])
        n45 = Build Array(w109) -> (w114:dbl[])
        n46 = Build Array(w108) -> (w116:dbl[])
        n47 = Build Array(w114, w116, w115) -> (w113:dbl[][])
        n48 = Transpose 2D Array(2D array=w113) -> (transposed array=→"Local Kalman Filters & Central Site Fusion":dbl[][])
      }
      frame Error {
        # "Sender did not send data. Ignore timeout error and keep waiting."
        n49 = Unbundle By Name(w125) -> ("code"=w126:i32)
        n50 = case shown="56" w126 {
          tunnel: w125 -> [w127 _]
          tunnel: [w127 w128] -> w124
          frame Default {
          }
          frame 56 {
            w128 = errorcluster {"status"=FALSE, "code"=0, "source"=""}  # No error
          }
        }
      }
    }
    n51 = node-c288(w91) -> ()  [unwired: 1 out]
  }
  n52 = disable-structure shown="Disabled" {
    frame Disabled {
      n53 = formula code="if(k < 660 || k > 710)\nyk = f;\nelse\nyk = k;"() -> ()  [unwired: 2 in, 1 out]
    }
    frame Enabled {
    }
  }
  n54 = disable-structure shown="Disabled" {
    frame Disabled {
      n55 = formula code="if(x < 600 || x > 710)\ny = f;\nelse\ny = x;"() -> ()  [unwired: 2 in, 1 out]
    }
    frame Enabled {
    }
  }
  n56 = node-c288(w65) -> (→"FPGA Loop Error":errorcluster)
  n57 = xnode "Close FPGA VI Reference"("FPGA VI Reference In"=w68, "error in"=w64) -> ("error out"=w63:errorcluster)
  n58 = Merge Errors(w63) -> (→"DAC Loop Error":errorcluster)
  n59 = node-c288(w54) -> (→"UDP Loop Error":errorcluster)
  n60 = node-c288(w2) -> (→"Error":errorcluster)
  n61 = UDP Close(connection ID=w61, 8:w59) -> (error out=w60:errorcluster)  [unwired: 1 out]
  n62 = call <vilib>:"Simple Error Handler.vi"("error in (no error)"=w60) -> ()  [unwired: 1 in, 8 out]
